vi "Data_get.vi"() -> ()   [LabVIEW 2009]
uses:
  <vilib>/Analysis/2dsp.llb/Real FFT.vi
  <vilib>/Analysis/NI_AALPro.lvlib
panel:
  in  "Repetition rate (Hz)":ext=2.5
  in  "Chirp start (MHz)":ext=2.5
  in  "Filter up to (MHz)":ext=2.5
  in  "Amount of averagings":u32
  out "Data":dbl[](array[numeric])
  out "XY Graph 5":cluster{ext[], dbl[]}(graph)
  out "FFT (Im)":dbl[](array[numeric])
  out "FFT (Re)":dbl[](array[numeric])
  out "Final array":ext[][](array[numeric])
  out "size(s)":i32
  in  "ns/div":u32
  in  "ps/point":u32
  out "Oscilloscope Data":dbl[](array[numeric])
  in  "Channel Number":u16=1
  out "Oscilloscope graph":dbl[](graph)
  in  "Stop":bool
  in  "TDS VISA Port":refnum<visa-resource-name>="GPIB0::1::INSTR"
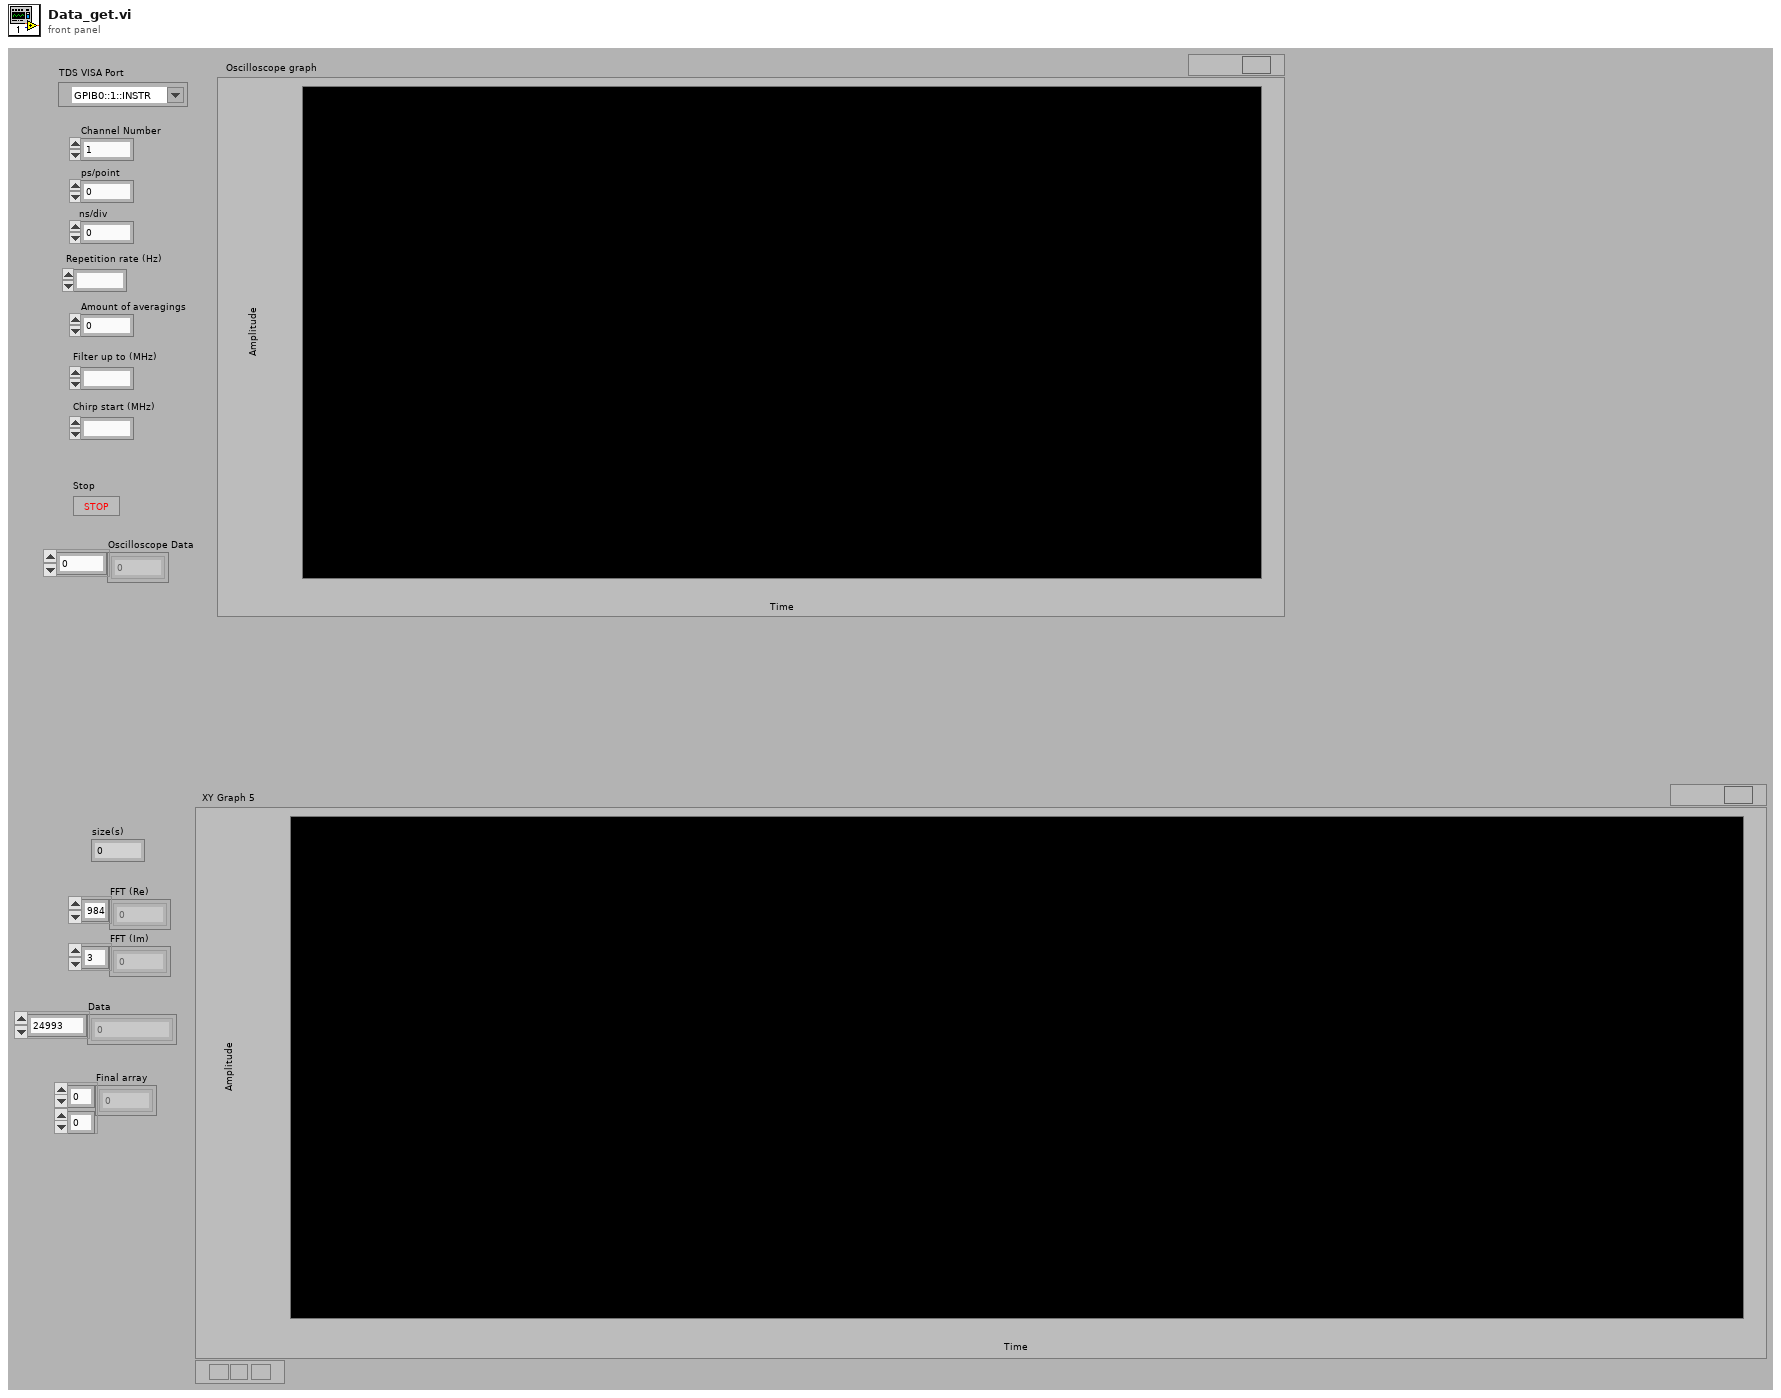
[diagram p1: front panel]
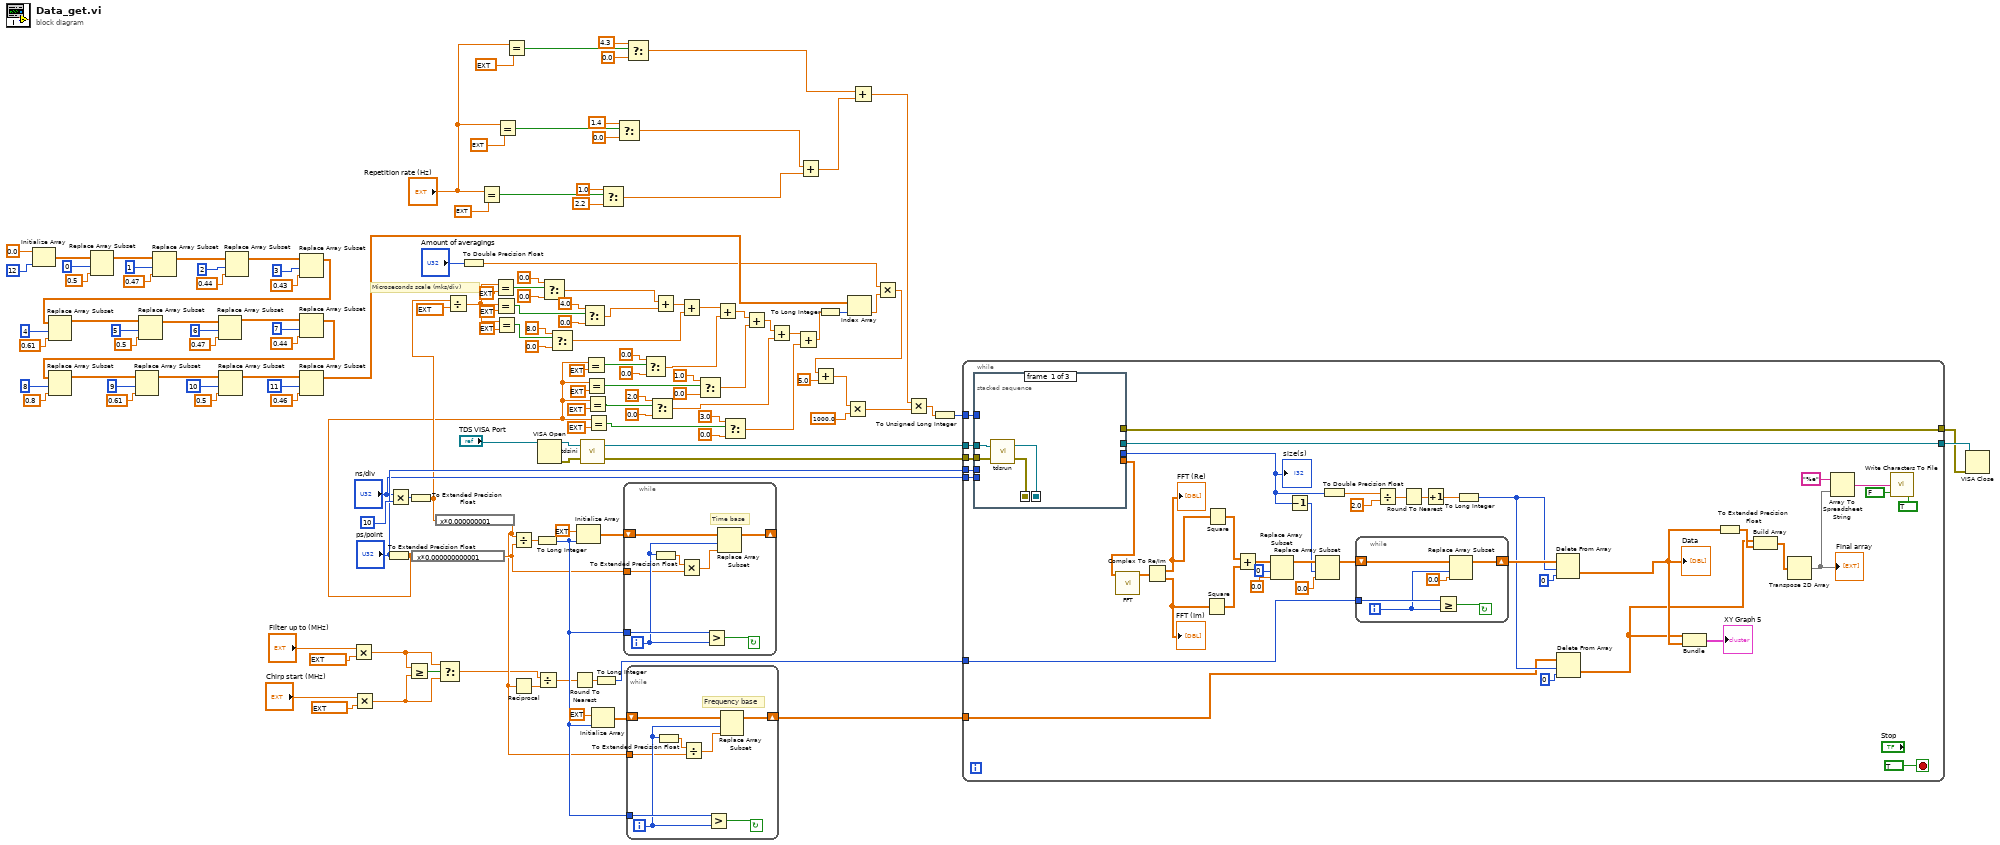
[diagram p0: block diagram]
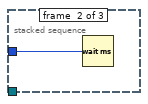
[diagram p2: hidden frame]
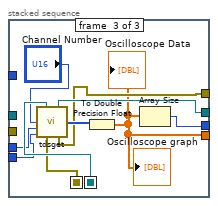
[diagram p3: hidden frame]
diagram:
  # "Microseconds scale (mks/div)"
  n1 = Initialize Array(0.0 ("element"), 12 ("dimension size")) -> (w121:dbl[])
  n2 = Replace Array Subset(array=w121, new element=0.5 ("new element/subarray"), index=0) -> (w116:dbl[])
  n3 = Replace Array Subset(array=w116, new element=0.47 ("new element/subarray"), index=1) -> (w95:dbl[])
  n4 = Replace Array Subset(array=w95, new element=0.44 ("new element/subarray"), index=2) -> (w94:dbl[])
  n5 = Replace Array Subset(array=w94, new element=0.43 ("new element/subarray"), index=3) -> (w93:dbl[])
  n6 = Replace Array Subset(array=w93, new element=0.61 ("new element/subarray"), index=4) -> (w92:dbl[])
  n7 = Replace Array Subset(array=w92, new element=0.5 ("new element/subarray"), index=5) -> (w91:dbl[])
  n8 = Replace Array Subset(array=w91, new element=0.47 ("new element/subarray"), index=6) -> (w90:dbl[])
  n9 = Replace Array Subset(array=w90, new element=0.44 ("new element/subarray"), index=7) -> (w89:dbl[])
  n10 = Replace Array Subset(array=w89, new element=0.8 ("new element/subarray"), index=8) -> (w88:dbl[])
  n11 = Replace Array Subset(array=w88, new element=0.61 ("new element/subarray"), index=9) -> (w87:dbl[])
  n12 = Replace Array Subset(array=w87, new element=0.5 ("new element/subarray"), index=10) -> (w86:dbl[])
  n13 = Replace Array Subset(array=w86, new element=0.46 ("new element/subarray"), index=11) -> (w44:dbl[])
  n14 = Multiply(x="Filter up to (MHz)", y=ext 1000000.0) -> (x*y=w24:ext)
  n15 = Multiply(x="Chirp start (MHz)", y=ext 1000000.0) -> (x*y=w21:ext)
  n16 = To Extended Precision Float(1:"ps/point") -> (0:w37:ext)
  n17 = Multiply(x="ns/div", y=u32 10) -> (x*y=w137:u32)
  n18 = Greater Or Equal?(x=w24, y=w21) -> (x >= y?=w33:bool)
  n19 = To Extended Precision Float(1:w137) -> (0:w125:ext)
  n20 = expression code="x*0.000000000001"(w37) -> (w126:ext)
  n21 = expression code="x*0.000000001"(w125) -> (w32:ext)
  n22 = Select(t=w24, s=w33, f=w21) -> (s? t:f=w30:ext)
  n23 = Divide(x=w125, y=ext 10000.0) -> (x/y=w85:ext)
  n24 = To Double Precision Float(number="Amount of averagings") -> (double precision float=w40:dbl)
  n25 = Equal?(x="Repetition rate (Hz)", y=ext 2.5) -> (x = y?=w19:bool)
  n26 = Equal?(x=w85, y=ext 1.0) -> (x = y?=w77:bool)
  n27 = Equal?(x=w85, y=ext 2.0) -> (x = y?=w72:bool)
  n28 = Equal?(x=w85, y=ext 4.0) -> (x = y?=w69:bool)
  n29 = Equal?(x="Repetition rate (Hz)", y=ext 0.5) -> (x = y?=w13:bool)
  n30 = Equal?(x="Repetition rate (Hz)", y=ext 0.25) -> (x = y?=w7:bool)
  n31 = Divide(x=w32, y=w126) -> (x/y=w136:ext)
  n32 = Reciprocal(x=w32) -> (1/x=w31:ext)
  n33 = To Long Integer(number=w136) -> (32bit integer=w128:i32)
  n34 = Divide(x=w30, y=w31) -> (x/y=w29:ext)
  n35 = VISA Open(VISA resource name="TDS VISA Port") -> (VISA resource name=w142:refnum<visa-resource-name>, error out=w143:errorcluster)  [unwired: 4 in]
  n36 = Select(t=0.0, s=w77, f=0.0) -> (s? t:f=w56:dbl)
  n37 = Select(t=8.0, s=w69, f=0.0) -> (s? t:f=w53:dbl)
  n38 = Round To Nearest(number=w29) -> (nearest integer value=w28:ext)
  n39 = Initialize Array(ext 0.0 ("element"), w128) -> (w132:ext[])
  n40 = call "tdsini.vi"("Error In (No Error)"=w143, "VISA Port In"=w142) -> ("Error Out"=w144:errorcluster, "VISA Port Out"=w145:refnum<visa-resource-name>)
  n41 = Select(t=4.0, s=w72, f=0.0) -> (s? t:f=w55:dbl)
  n42 = Equal?(x=w37, y=ext 25.0) -> (x = y?=w60:bool)
  n43 = Equal?(x=w37, y=ext 50.0) -> (x = y?=w59:bool)
  n44 = Equal?(x=w37, y=ext 100.0) -> (x = y?=w58:bool)
  n45 = Equal?(x=w37, y=ext 200.0) -> (x = y?=w57:bool)
  n46 = Initialize Array(ext 0.0 ("element"), w128) -> (w130:ext[])
  n47 = To Long Integer(number=w28) -> (32bit integer=w27:i32)
  n48 = Select(t=1.0, s=w19, f=2.2) -> (s? t:f=w9:dbl)
  n49 = Select(t=1.4, s=w13, f=0.0) -> (s? t:f=w10:dbl)
  n50 = while {
    tunnel: w128 -> [w152]
    shift-right: [w150] -> _
    shift-left: w132 -> [w151]
    tunnel: w126 -> [w147]
    i -> [w149]
    stop <- w153 continue-if-true
    # "Time base"
    n51 = To Extended Precision Float(1:w149) -> (0:w148:ext)
    n52 = Multiply(x=w148, y=w147) -> (x*y=w146:ext)
    n53 = Greater?(x=w152, y=w149) -> (0:w153:bool)
    n54 = Replace Array Subset(array=w151, new element=w146, index=w149) -> (w150:ext[])
  }
  n55 = Select(t=4.3, s=w7, f=0.0) -> (s? t:f=w3:dbl)
  n56 = while {
    tunnel: w128 -> [w160]
    shift-right: [w158] -> w129
    shift-left: w130 -> [w159]
    tunnel: w32 -> [w155]
    i -> [w157]
    stop <- w161 continue-if-true
    # "Frequency base"
    n57 = To Extended Precision Float(1:w157) -> (0:w156:ext)
    n58 = Divide(x=w156, y=w155) -> (x/y=w154:ext)
    n59 = Greater?(x=w160, y=w157) -> (0:w161:bool)
    n60 = Replace Array Subset(array=w159, new element=w154, index=w157) -> (w158:ext[])
  }
  n61 = Select(t=0.0, s=w60, f=0.0) -> (s? t:f=w51:dbl)
  n62 = Select(t=2.0, s=w58, f=0.0) -> (s? t:f=w47:dbl)
  n63 = Add(x=w56, y=w55) -> (x+y=w54:dbl)
  n64 = Add(x=w54, y=w53) -> (x+y=w52:dbl)
  n65 = Select(t=1.0, s=w59, f=0.0) -> (s? t:f=w49:dbl)
  n66 = Add(x=w52, y=w51) -> (x+y=w50:dbl)
  n67 = Select(t=3.0, s=w57, f=0.0) -> (s? t:f=w45:dbl)
  n68 = Add(x=w50, y=w49) -> (x+y=w48:dbl)
  n69 = Add(x=w48, y=w47) -> (x+y=w46:dbl)
  n70 = Add(x=w46, y=w45) -> (x+y=w42:dbl)
  n71 = Add(x=w10, y=w9) -> (x+y=w2:dbl)
  n72 = To Long Integer(number=w42) -> (32bit integer=w43:i32)
  n73 = Index Array(array=w44, index=w43) -> (element=w41:dbl)
  n74 = Add(x=w3, y=w2) -> (x+y=w1:dbl)
  n75 = Multiply(x=w40, y=w41) -> (x*y=w36:dbl)
  n76 = Add(x=w36, y=5.0) -> (x+y=w34:dbl)
  n77 = Multiply(x=w34, y=1000.0) -> (x*y=w16:dbl)
  n78 = Multiply(x=w1, y=w16) -> (x*y=w15:dbl)
  n79 = To Unsigned Long Integer(number=w15) -> (unsigned 32bit integer=w38:u32)
  n80 = while {
    tunnel: [w201] -> w139
    tunnel: [w202] -> w140
    tunnel: w144 -> [w203]
    tunnel: w145 -> [w204]
    tunnel: "ps/point" -> [w200]
    tunnel: "ns/div" -> [w199]
    tunnel: w129 -> [w163]
    tunnel: w38 -> [w180]
    tunnel: w27 -> [w176]
    stop <- TRUE stop-if-true
    n81 = stacked-sequence {
      seq-local: [w212 _ _] -> [_ _ w225]
      seq-local: [w211 _ _] -> [_ _ w218]
      tunnel: w204 -> [w213 _ _]
      tunnel: w203 -> [w214 _ _]
      tunnel: [_ _ w223] -> w202
      tunnel: [_ _ w222] -> w201
      tunnel: w200 -> [_ _ w220]
      tunnel: w199 -> [_ _ w219]
      tunnel: [_ _ w217] -> w174
      tunnel: [_ _ w216] -> w192
      tunnel: w180 -> [_ w215 _]
      frame #0 {
        n82 = call "tdsrun.vi"("Error In (No Error)"=w214, "VISA Port In"=w213) -> ("Error Out"=w211:errorcluster, "VISA Port Out"=w212:refnum<visa-resource-name>)
      }
      frame #1 {
        n83 = Wait (ms)(milliseconds to wait=w215) -> ()  [unwired: 1 out]
      }
      frame #2 {
        n84 = call "tdsget.vi"("VISA Port In"=w225, "Channel Number"="Channel Number", "ps/point"=w220, "ns/div"=w219, "Error In (No Error)"=w218) -> ("VISA Port Out"=w223:refnum<visa-resource-name>, "TDS Data"=w224:u16[], "Error Out"=w222:errorcluster)  [unwired: 8 in]
        n85 = To Double Precision Float(number=w224) -> (double precision float=w216:dbl[])
        "Oscilloscope graph" <- w216
        "Oscilloscope Data" <- w216
        n86 = Array Size(array=w216) -> (size(s)=w217:i32)
      }
    }
    "size(s)" <- w174
    n87 = call-poly <vilib>:"FFT.vi"("X"=w192) -> ("FFT {X}"=w198:cdb[])  [unwired: 9 in, 1 out]
    n88 = Complex To Re/Im(x + iy=w198) -> (x=w197:dbl[], y=w196:dbl[])
    "FFT (Re)" <- w197
    "FFT (Im)" <- w196
    n89 = Square(x=w196) -> (x^2=w194:dbl[])
    n90 = Square(x=w197) -> (x^2=w195:dbl[])
    n91 = Add(x=w195, y=w194) -> (x+y=w184:dbl[])
    n92 = Replace Array Subset(array=w184, new element=0.0 ("new element/subarray"), index=0) -> (w183:dbl[])
    n93 = Decrement(x=w174) -> (x-1=w182:i32)
    n94 = Replace Array Subset(array=w183, new element=0.0 ("new element/subarray"), index=w182) -> (w177:dbl[])
    n95 = To Double Precision Float(number=w174) -> (double precision float=w173:dbl)
    n96 = while {
      tunnel: w176 -> [w209]
      shift-right: [w207] -> w175
      shift-left: w177 -> [w208]
      i -> [w206]
      stop <- w210 continue-if-true
      n97 = Greater Or Equal?(x=w209, y=w206) -> (x >= y?=w210:bool)
      n98 = Replace Array Subset(array=w208, new element=0.0 ("new element/subarray"), index=w206) -> (w207:dbl[])
    }
    n99 = Divide(x=w173, y=2.0) -> (x/y=w171:dbl)
    n100 = Round To Nearest(number=w171) -> (nearest integer value=w170:dbl)
    n101 = Increment(x=w170) -> (x+1=w169:dbl)
    n102 = To Long Integer(number=w169) -> (32bit integer=w164:i32)
    n103 = Delete From Array(array=w175, length=w164, index=0) -> (deleted portion=w167:dbl[])  [unwired: 1 out]
    "Data" <- w167
    n104 = Delete From Array(array=w163, length=w164, index=0) -> (deleted portion=w162:ext[])  [unwired: 1 out]
    n105 = Bundle(w162, w167) -> (→"XY Graph 5":cluster{ext[], dbl[]})  [unwired: 1 in]
    n106 = To Extended Precision Float(1:w167) -> (0:w166:ext[])
    n107 = Build Array(w162, w166) -> (w178:ext[][])
    n108 = Transpose 2D Array(2D array=w178) -> (transposed array=w190:ext[][])
    "Final array" <- w190
    n109 = Array To Spreadsheet String(array=w190, 3:"%e") -> (spreadsheet string=w187:string)  [unwired: 1 in]
    n110 = call <vilib>:"Write Characters To File.vi"("convert eol? (no:F)"=TRUE, "append to file? (new file:F)"=FALSE, "character string"=w187) -> ()  [unwired: 2 in, 1 out]
  }
  n111 = VISA Close(VISA resource name=w140, error in (no error)=w139) -> ()  [unwired: 1 out]
